vi "Aquisicao_UDP_paralelo.vi"(1 "file path (dialog if empty)":path, 2 "mode":i32=1, 3 "Tempo Aquisicao":dbl, 4 "reference in":refnum<vi>) -> ()   [LabVIEW 2019]
uses:
  <vilib>/Utility/file.llb/Read Delimited Spreadsheet (string).vi
  <vilib>/Utility/file.llb/Write Delimited Spreadsheet (string).vi
  <vilib>/Utility/file.llb/Write Delimited Spreadsheet (DBL).vi
panel:
  out "modo de retirada":string
  out "Jw":dbl[](array[numeric])
  out "Jk":dbl[](array[numeric])
  out "TimeStamp string":string
  out "Quantidade de pontos":i32
  out "Recebendo velocidades":bool
  out "Array_velocidades":dbl[][](array[numeric]) format="%#_30g"
  out "reference out":refnum<vi>
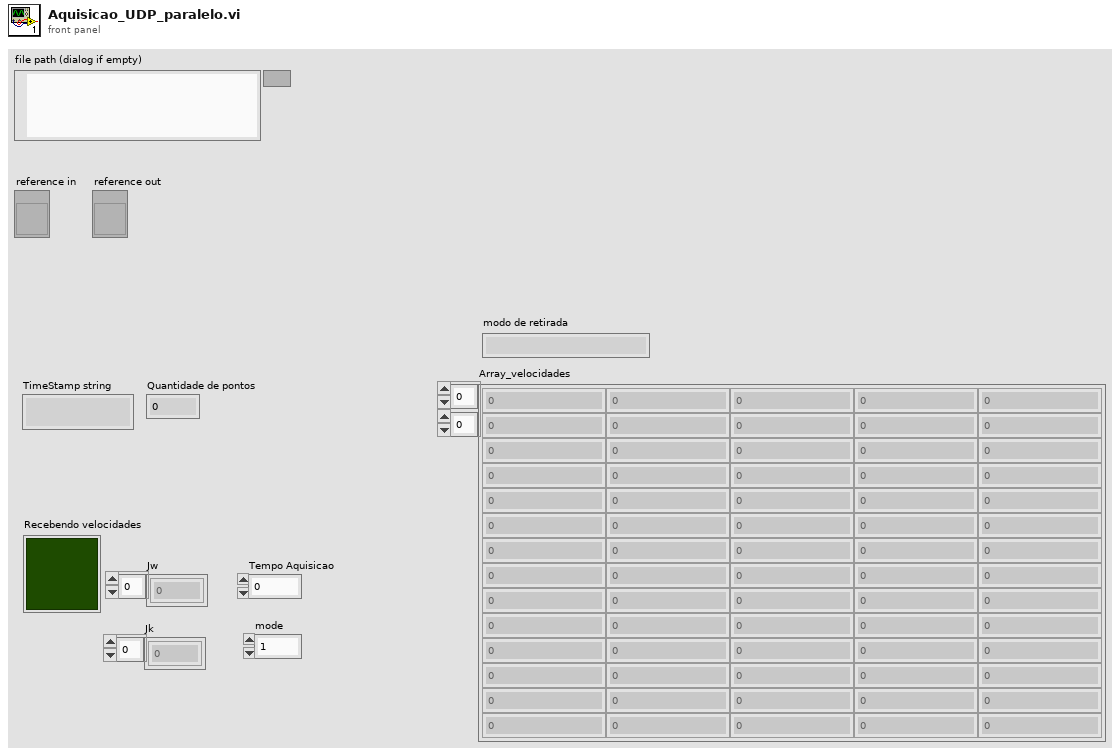
[diagram p1: front panel]
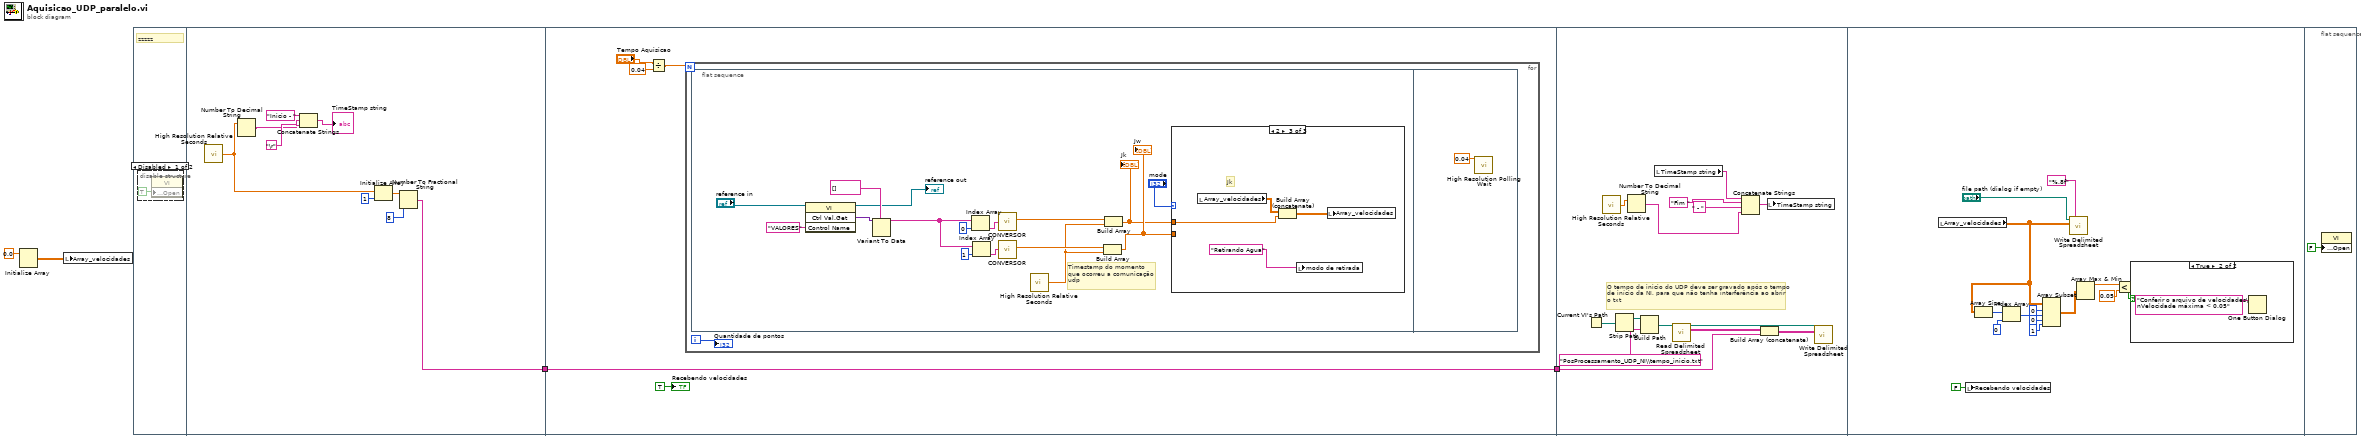
[diagram p0: block diagram]
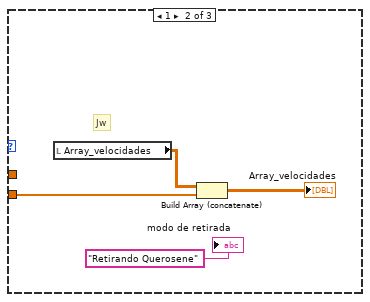
[diagram p4: hidden frame]
diagram:
  n1 = Initialize Array(0.0 ("element")) -> (w3:dbl[][])  [unwired: 2 in]
  n2 = local write "Array_velocidades"(w3) -> ()
  n3 = flat-sequence {
    tunnel: [w8] -> w1
    tunnel: [w18] -> w2
    tunnel: w1 -> [w18]
    tunnel: w2 -> [w49]
    frame #0 {
      # "zzzzz"
      n4 = disable-structure shown="Disabled" {
        frame Disabled {
          n5 = property class="VI"("Front Panel.Open"=TRUE ("Front Panel Window:Open")) -> ()  [unwired: 2 in, 2 out]
        }
        frame Enabled {
        }
      }
    }
    frame #1 {
      n6 = call <vilib>:"High Resolution Relative Seconds.vi"() -> ("relative seconds"=w6:dbl)
      n7 = Number To Decimal String(number=w6) -> (decimal integer string=w7:string)  [unwired: 1 in]
      n8 = Concatenate Strings("Inicio - " ("string"), w7, "\r") -> (→"TimeStamp string":string)
      n9 = Initialize Array(w6, 1 ("dimension size")) -> (w10:dbl[])
      n10 = Number To Fractional String(number=w10, precision (6)=i16 8) -> (F-format string=w8:string[])  [unwired: 2 in]
    }
    frame #2 {
      n11 = Divide(x="Tempo Aquisicao", y=0.04) -> (x/y=w16:dbl)
      n12 = for {
        N: w16 -> [_]
        i -> [w20]
        n13 = flat-sequence {
          frame #0 {
            # "Timestamp do momento\nque ocorreu a comunicação\nudp"
            n14 = invoke class="VI" method="Ctrl Val.Get"(reference="reference in", "Control Name"="VALORES") -> (reference out=→"reference out":refnum<vi>, "Get Control Value Variant"=w28:variant)  [unwired: 2 in, 2 out]
            n15 = Variant To Data(type=string[] [] ("Array"), Variant=w28) -> (data=w23:string[])  [unwired: 1 in, 1 out]
            n16 = Index Array(array=w23, index=0) -> (element=w22:string)
            n17 = Index Array(array=w23, index=1) -> (element=w21:string)
            n18 = call "CONVERSOR.vi"("String"=w22) -> ("float"=w33:dbl)  [unwired: 6 in, 3 out]
            n19 = call "CONVERSOR.vi"("String"=w21) -> ("float"=w35:dbl)  [unwired: 6 in, 3 out]
            n20 = call <vilib>:"High Resolution Relative Seconds.vi"() -> ("relative seconds"=w31:dbl)
            n21 = Build Array(w35, w31) -> (w34:dbl[])
            "Jw" <- w34
            n22 = Build Array(w33, w31) -> (w32:dbl[])
            "Jk" <- w32
            n23 = case shown="2" "mode" {
              tunnel: w32 -> [_ _ w43]
              tunnel: w34 -> [_ w38 _]
              frame 0, Default {
              }
              frame 1 {
                # "Jw"
                n24 = local read "Array_velocidades"() -> (w39:dbl[][])
                n25 = Build Array (concatenate)(w39, w38) -> (→"Array_velocidades":dbl[][])
                "modo de retirada" <- "Retirando Querosene" ("modo de retirada")
              }
              frame 2 {
                # "Jk"
                n26 = local read "Array_velocidades"() -> (w44:dbl[][])
                n27 = Build Array (concatenate)(w44, w43) -> (w42:dbl[][])
                n28 = local write "modo de retirada"("Retirando Agua" ("modo de retirada")) -> ()
                n29 = local write "Array_velocidades"(w42) -> ()
              }
            }
          }
          frame #1 {
            n30 = call <vilib>:"High Resolution Polling Wait.vi"("seconds to wait"=0.04) -> ()  [unwired: 10 in, 1 out]
          }
        }
        "Quantidade de pontos" <- w20
      }
      "Recebendo velocidades" <- TRUE ("Recebendo velocidades")
    }
    frame #3 {
      # "O tempo de inicio do UDP deve ser gravado após o tempo\nde início da NI, para que não tenha interferência ao abrir\no txt"
      n31 = Current VI's Path() -> (path=w51:path)
      n32 = call <vilib>:"High Resolution Relative Seconds.vi"() -> ("relative seconds"=w47:dbl)
      n33 = Strip Path(path=w51) -> (stripped path=w50:path)  [unwired: 1 out]
      n34 = Number To Decimal String(number=w47) -> (decimal integer string=w46:string)  [unwired: 1 in]
      n35 = Build Path(base path=w50, name or relative path="PosProcessamento_UDP_NI\\tempo_inicio.txt") -> (appended path=w53:path)
      n36 = local read "TimeStamp string"() -> (w56:string)
      n37 = call-poly <vilib>:"Read Delimited Spreadsheet.vi"("file path (dialog if empty)"=w53) -> ("new file path (Not A Path if cancelled)"=w55:path, "all rows"=w52:string[][])  [unwired: 9 in, 4 out]
      n38 = Concatenate Strings(w56, "Fim " ("string"), " - " ("string"), w46) -> (w57:string)
      n39 = Build Array (concatenate)(w52, w49) -> (w54:string[][])
      n40 = local write "TimeStamp string"(w57) -> ()
      n41 = call-poly <vilib>:"Write Delimited Spreadsheet.vi"("file path (dialog if empty)"=w55, "2D data"=w54) -> ()  [unwired: 12 in, 2 out]
    }
    frame #4 {
      n42 = local read "Array_velocidades"() -> (w63:dbl[][])
      n43 = local write "Recebendo velocidades"(FALSE ("Recebendo velocidades")) -> ()
      n44 = Array Size(array=w63) -> (size(s)=w62:i32[])
      n45 = Index Array(array=w62, index=0) -> (element=w60:i32)
      n46 = Array Subset(array=w63, index (row)=0 ("index"), length (row)=w60, index (col)=0 ("index"), length (col)=1 ("length")) -> (w67:dbl[][])
      n47 = call-poly <vilib>:"Write Delimited Spreadsheet.vi"("file path (dialog if empty)"="file path (dialog if empty)", "format (%.3f)"="%.8f", "2D data"=w63) -> ()  [unwired: 11 in, 2 out]
      n48 = Array Max & Min(array=w67) -> (max value=w70:dbl)  [unwired: 3 out]
      n49 = Less?(x=w70, y=0.05) -> (x < y?=w68:bool)
      n50 = case shown="True" w68 {
        frame False {
        }
        frame True {
          n51 = One Button Dialog(message="Conferir o arquivo de velocidades\nVelocidade máxima < 0.05") -> ()  [unwired: 1 in, 1 out]
        }
      }
    }
    frame #5 {
      n52 = property class="VI"("Front Panel.Open"=FALSE ("Front Panel Window:Open")) -> ()  [unwired: 2 in, 2 out]
    }
  }
